vi "ErrorCodeToErrorInfo.vi"(8 "return type":u8) -> (0 "StatusInfo":T1)   [LabVIEW 2016, in "fgt_SDK.lvlib"]
uses:
  fgt_SDK.lvlib
  TypeDefs/fgt_INSTRUMENT_TYPE.ctl
  TypeDefs/fgt_STATUS_INFO.ctl
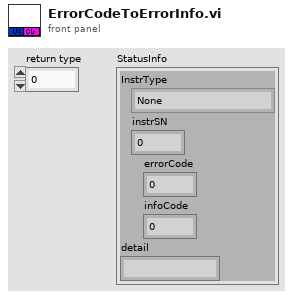
[diagram p1: front panel]
types:
  T1 = typedef "fgt_SDK.lvlib/fgt_STATUS_INFO.ctl" = cluster{"InstrType":T2, "instrSN":u16, "errorCode":u8, "infoCode":u8, "detail":string}
  T2 = typedef "fgt_SDK.lvlib/fgt_INSTRUMENT_TYPE.ctl" = enum32{"None", "MFCS", "MFCS_EZ", "FRP", "LineUP", "IPS"}
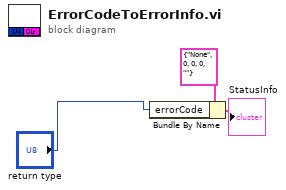
[diagram p0: block diagram]
diagram:
  n1 = Bundle By Name(cluster=T1 {"InstrType"=enum."None", "instrSN"=0, "errorCode"=0, "infoCode"=0, "detail"=""} ("StatusInfo"), "errorCode"="return type") -> (→"StatusInfo":T1)
